vi "audio-stim.vi"() -> ()   [LabVIEW 2009]
panel:
  in  "Stimulus List Start Num":i32 caption="Stimulus List Numbering Start"
  in  "stop":bool
  in  "Save Stimulus List":bool
  in  "Load Parameter List":bool
  in  "Save Parameter List":bool
  in  "Repetitions":i32 caption="# of Random Repetitions for Each Stimulus" min=2
  in  "Parameter List":dbl[][](array[numeric])
  out "Stimulus List":dbl[][](array[numeric])
  in  "Load Stimulus List":bool
  out "Stimulus List Path":path
  out "Parameter Path":path
  in  "Play":bool
  in  "Generate Stimulus List":bool
  # "Stim Type, Duration, Amplitude, Param 1, Param 2, Param 3, Param 4"
  # "Stim#, Stim Type, Duration, Amplitude, Param 1, Param 2, Param 3, Param 4"
  # "Stim Type 1 DC (no parameters, just amplitude)"
  # "Stim Type 3 Pure Tone (param1 = frequency)"
  # "Stim Type 4 FM Sweep (param1 = start frequency, param2 = end frequency)"
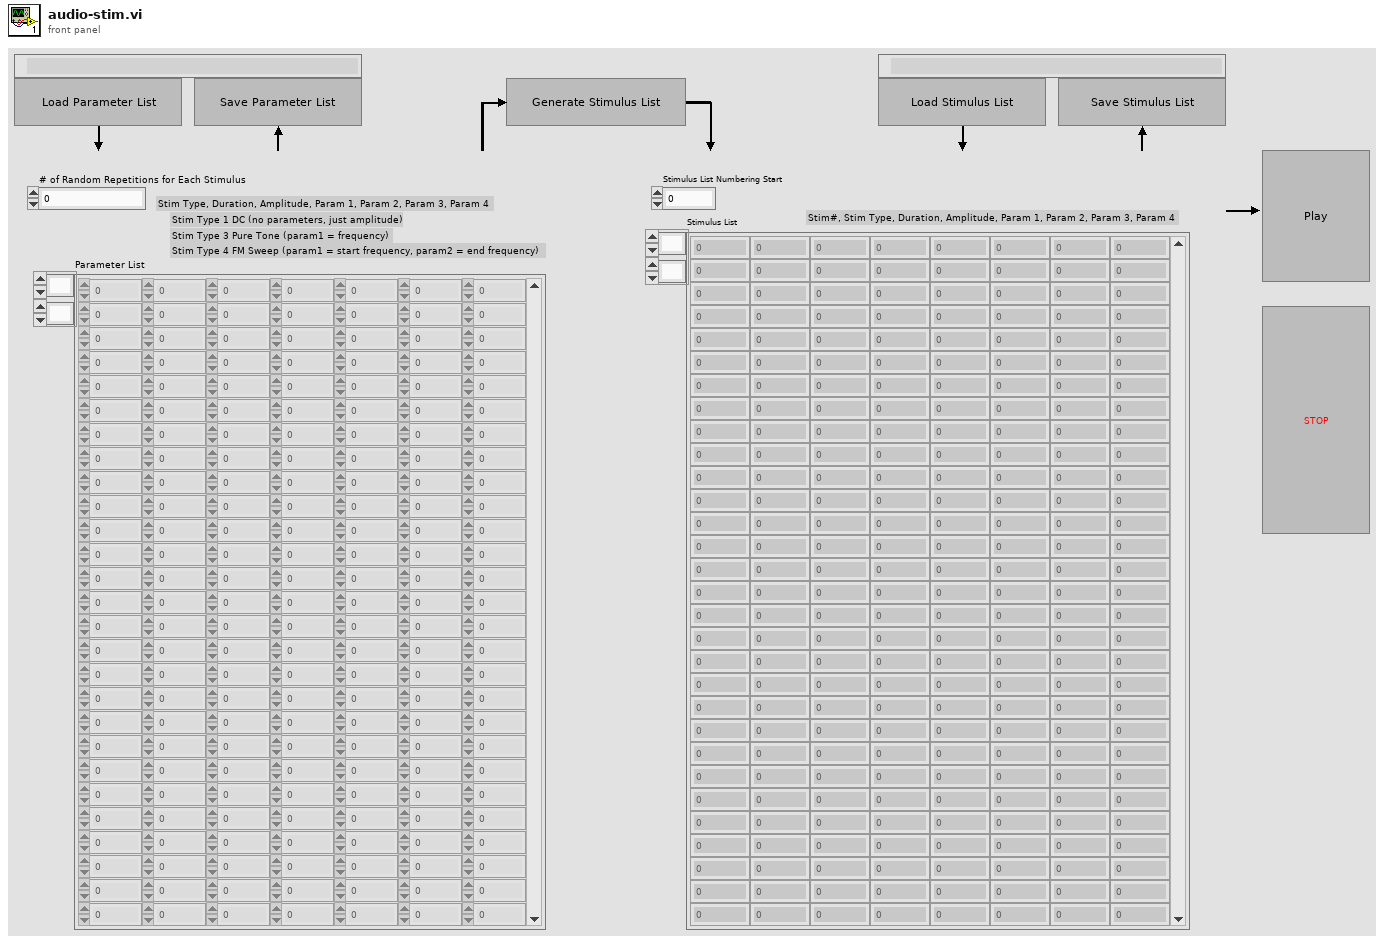
[diagram p1: front panel]
types:
  T1 = enum8{"Enabled", "Disabled", "Disabled and Grayed Out"}
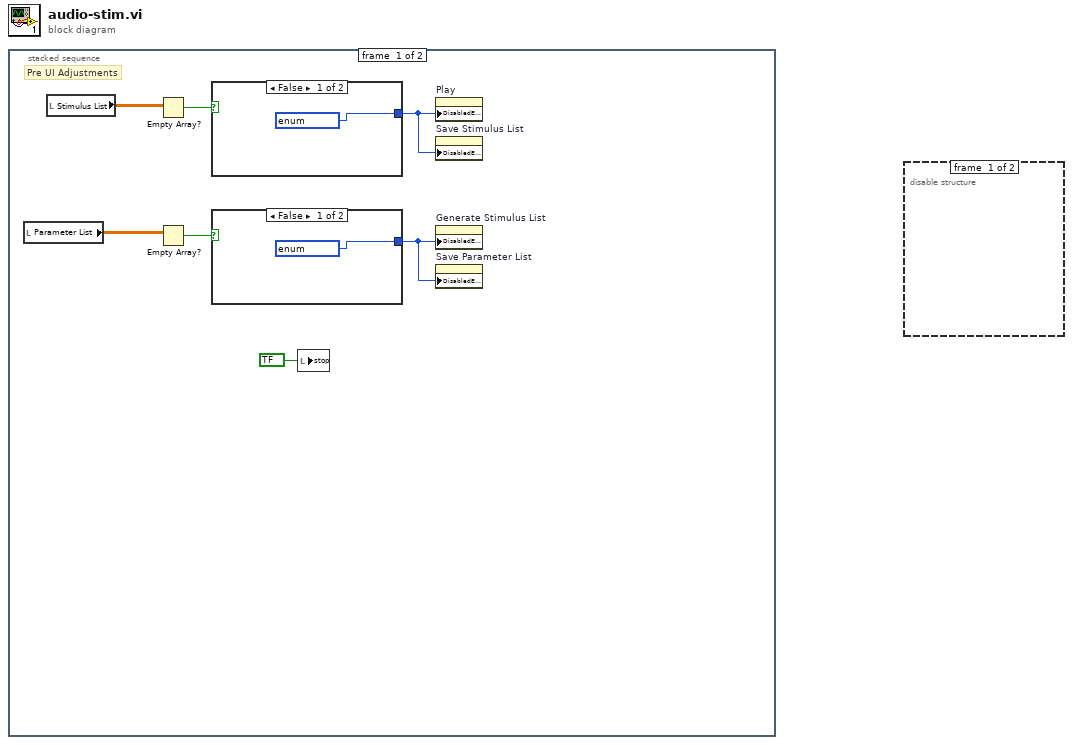
[diagram p0: block diagram]
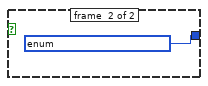
[diagram p3: hidden frame]
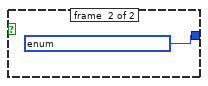
[diagram p4: hidden frame]
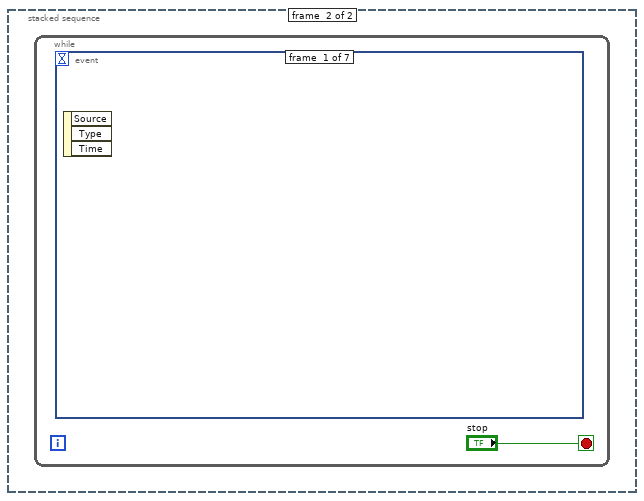
[diagram p5: hidden frame]
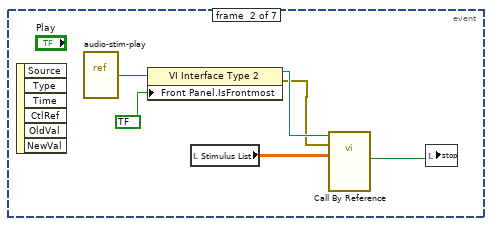
[diagram p6: hidden frame]
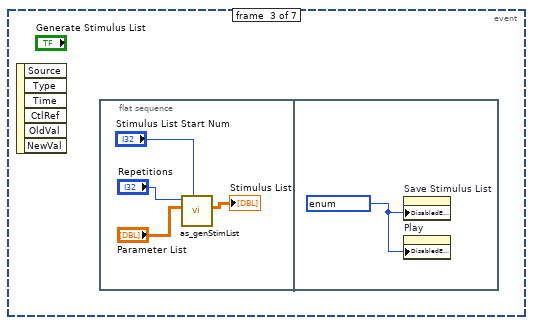
[diagram p7: hidden frame]
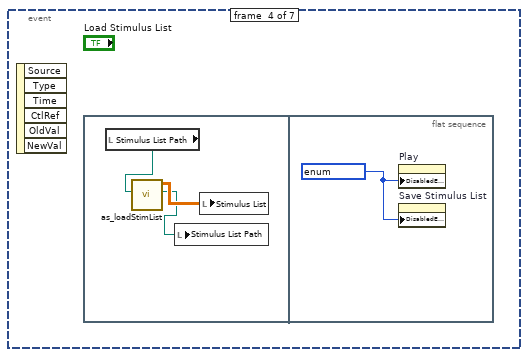
[diagram p8: hidden frame]
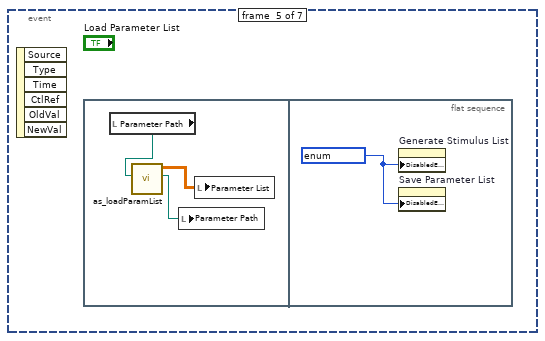
[diagram p9: hidden frame]
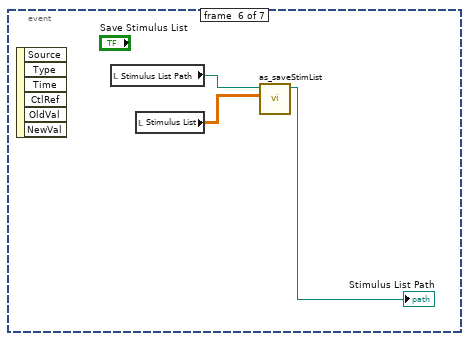
[diagram p10: hidden frame]
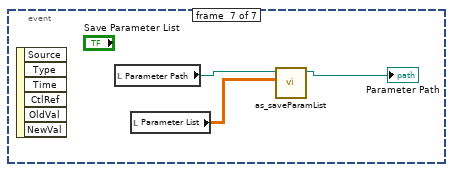
[diagram p11: hidden frame]
diagram:
  n1 = stacked-sequence {
    frame #0 {
      # "Pre UI Adjustments"
      n2 = local read "Parameter List"() -> (w2:dbl[][])
      n3 = local read "Stimulus List"() -> (w7:dbl[][])
      n4 = Empty Array?(array=w7) -> (empty?=w6:bool)
      n5 = Empty Array?(array=w2) -> (empty?=w4:bool)
      n6 = case shown="False" w6 {
        tunnel: [T1 ? ("Disabled") T1 ? ("Disabled")] -> w5
        frame #0 {
        }
        frame #1 {
        }
      }
      n7 = case shown="False" w4 {
        tunnel: [T1 ? ("Disabled") T1 ? ("Disabled")] -> w3
        frame #0 {
        }
        frame #1 {
        }
      }
      n8 = local write "stop"(bool ? ("stop")) -> ()
      n9 = property on="Play" class="Bool (strict)"("DisabledEnum"=w5) -> ()  [unwired: 2 in, 2 out]
      n10 = property on="Save Stimulus List" class="Bool"("DisabledEnum"=w5) -> ()  [unwired: 2 in, 2 out]
      n11 = property on="Generate Stimulus List" class="Bool"("DisabledEnum"=w3) -> ()  [unwired: 2 in, 2 out]
      n12 = property on="Save Parameter List" class="Bool"("DisabledEnum"=w3) -> ()  [unwired: 2 in, 2 out]
    }
    frame #1 {
      n13 = while {
        stop <- "stop" stop-if-true
        n14 = event shown="[1] \"Play\": Value Change" {
          selector: _ -> [_ _ _ _ _ _ _]
          dyn-events: _ -> [_ _ _ _ _ _ _]
          timeout: _ -> [_ _ _ _ _ _ _]
          event #0 {
            n15 = event-data() -> ()  [unwired: 1 in, 3 out]
          }
          event #1 {
            n16 = event-data() -> ()  [unwired: 1 in, 6 out]
            n17 = vi-ref "audio-stim-play.vi"() -> (w18:refnum<vi>)
            n18 = property class="VI Interface Type 2"(reference=w18, "Front Panel.IsFrontmost"=bool ? ("Execution:Show Front Panel On Call")) -> (reference out=w15:refnum<vi>, error out=w14:errorcluster)  [unwired: 1 in]
            n19 = local read "Stimulus List"() -> (w16:dbl[][])
            n20 = call-by-ref "?"(reference=w15, error in=w14, "Stimulus List"=w16) -> ("Playing"=w13:bool)  [unwired: 10 in, 2 out]
            n21 = local write "stop"(w13) -> ()
          }
          event #2 {
            n22 = event-data() -> ()  [unwired: 1 in, 6 out]
            n23 = flat-sequence {
              frame #0 {
                n24 = call "as_genStimList.vi"("Stimulus List Start Num"="Stimulus List Start Num", "Stimulus Parameters"="Parameter List", "Repetitions"="Repetitions") -> ("Stimulus List"=→"Stimulus List":dbl[][])  [unwired: 8 in]
              }
              frame #1 {
                w23 = T1 ? ("Disabled")
                n25 = property on="Save Stimulus List" class="Bool"("DisabledEnum"=w23) -> ()  [unwired: 2 in, 2 out]
                n26 = property on="Play" class="Bool (strict)"("DisabledEnum"=w23) -> ()  [unwired: 2 in, 2 out]
              }
            }
          }
          event #3 {
            n27 = event-data() -> ()  [unwired: 1 in, 6 out]
            n28 = flat-sequence {
              frame #0 {
                n29 = local read "Stimulus List Path"() -> (w26:path)
                n30 = call "as_loadStimList.vi"("Path In"=w26) -> ("Path"=w24:path, "Stimulus List"=w25:dbl[][])  [unwired: 4 in, 1 out]
                n31 = local write "Stimulus List Path"(w24) -> ()
                n32 = local write "Stimulus List"(w25) -> ()
              }
              frame #1 {
                w27 = T1 ? ("Disabled")
                n33 = property on="Play" class="Bool (strict)"("DisabledEnum"=w27) -> ()  [unwired: 2 in, 2 out]
                n34 = property on="Save Stimulus List" class="Bool"("DisabledEnum"=w27) -> ()  [unwired: 2 in, 2 out]
              }
            }
          }
          event #4 {
            n35 = event-data() -> ()  [unwired: 1 in, 6 out]
            n36 = flat-sequence {
              frame #0 {
                n37 = local read "Parameter Path"() -> (w28:path)
                n38 = call "as_loadParamList.vi"("Path In"=w28) -> ("Path"=w29:path, "Stimulus List"=w30:dbl[][])  [unwired: 4 in, 1 out]
                n39 = local write "Parameter Path"(w29) -> ()
                n40 = local write "Parameter List"(w30) -> ()
              }
              frame #1 {
                w31 = T1 ? ("Disabled")
                n41 = property on="Generate Stimulus List" class="Bool"("DisabledEnum"=w31) -> ()  [unwired: 2 in, 2 out]
                n42 = property on="Save Parameter List" class="Bool"("DisabledEnum"=w31) -> ()  [unwired: 2 in, 2 out]
              }
            }
          }
          event #5 {
            n43 = event-data() -> ()  [unwired: 1 in, 6 out]
            n44 = local read "Stimulus List Path"() -> (w33:path)
            n45 = local read "Stimulus List"() -> (w32:dbl[][])
            n46 = call "as_saveStimList.vi"("Stimulus List"=w32, "Path In"=w33) -> ("Path"=→"Stimulus List Path":path)  [unwired: 4 in, 1 out]
          }
          event #6 {
            n47 = event-data() -> ()  [unwired: 1 in, 6 out]
            n48 = local read "Parameter Path"() -> (w37:path)
            n49 = local read "Parameter List"() -> (w35:dbl[][])
            n50 = call "as_saveParamList.vi"("Stimulus List"=w35, "Path In"=w37) -> ("Path"=→"Parameter Path":path)  [unwired: 4 in, 1 out]
          }
        }
      }
    }
  }
  n51 = disable-structure shown="Enabled" {
    frame #0 {
    }
    frame #1 {
    }
  }
